vi "Convert to Fahrenheit.vi"(1 "Celsius":dbl) -> (0 "Fahrenheit":dbl)   [LabVIEW 2019]
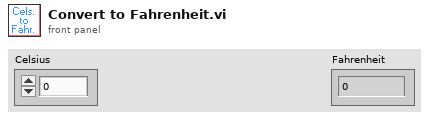
[diagram p1: front panel]
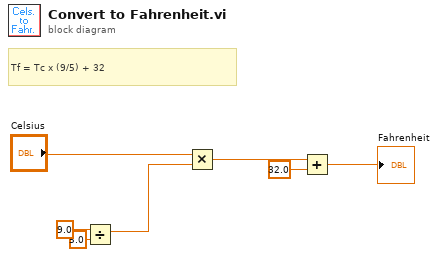
[diagram p0: block diagram]
diagram:
  # "Tf = Tc x (9/5) + 32"
  n1 = Divide(x=9.0, y=5.0) -> (x/y=w4:dbl)
  n2 = Multiply(x="Celsius", y=w4) -> (x*y=w3:dbl)
  n3 = Add(x=w3, y=32.0) -> (x+y=→"Fahrenheit":dbl)
